vi "Time_x_graph.vi"(0 "Inital array":dbl[](array[numeric]), 7 "Time inputs":dbl=1750.0, 11 "Timing control":i32=51) -> (4 "Array":i32[](array[numeric]), 8 "PW OUT":dbl, 14 "Boolean 2":bool, 15 "N points":i32=51)   [LabVIEW 2019]
doc: "This subvi produce the x componant of our xy graph which is the timing portion of the graph. \nalso it does true false if we have valid PW out input"
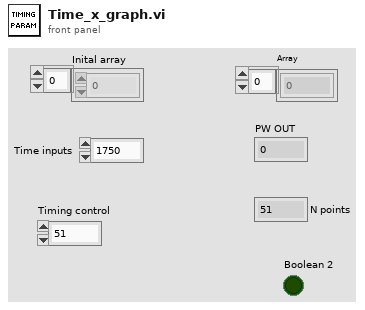
[diagram p1: front panel]
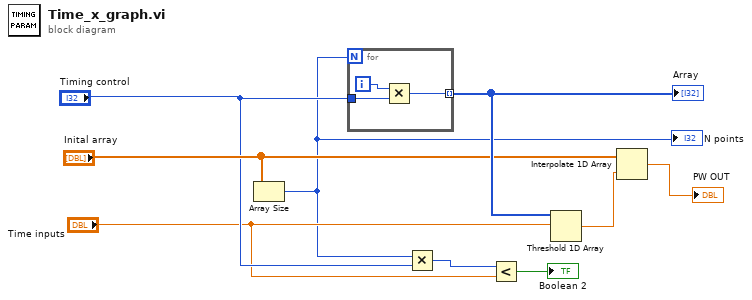
[diagram p0: block diagram]
diagram:
  n1 = Array Size(array="Inital array") -> (size(s)=w1:i32)
  "N points" <- w1
  n2 = for {
    N: w1 -> [_]
    tunnel: "Timing control" -> [w11]
    tunnel: [w10] -> w8 mode=indexing
    i -> [w12]
    n3 = Multiply(x=w12, y=w11) -> (x*y=w10:i32)
  }
  "Array" <- w8
  n4 = Multiply(x=w1, y="Timing control") -> (x*y=w3:i32)
  n5 = Less?(x=w3, y="Time inputs") -> (x < y?=→"Boolean 2":bool)
  n6 = Threshold 1D Array(2:"Time inputs", 3:w8) -> (0:w4:dbl)  [unwired: 1 in]
  n7 = Interpolate 1D Array(1:w4, 2:"Inital array") -> (0:→"PW OUT":dbl)
